vi "CSTK_BuildApplication_Manager_RenameEXEFileName.vi"(8 "错误输入（无错误）":errorcluster, 11 "BuildApplication Data in":T1={"Build Specification Name"="", "Destination Path"=path "", "Files Generated by Build"=[], "Exe Path Generated by Build"=path "", "Version"="", "Datatime"=timestamp(0 s since 1904-01-01), "ChangeLog"="", "Package as a ZIP file?"=TRUE, "Rename EXE File Name?"=FALSE, "Zip File Path"=path ""} {"Datatime" format="%<%.3X %x>T"}) -> (0 "错误输出":errorcluster, 3 "BuildApplication Data out":T1={"Build Specification Name"="", "Destination Path"=path "", "Files Generated by Build"=[], "Exe Path Generated by Build"=path "", "Version"="", "Datatime"=timestamp(0 s since 1904-01-01), "ChangeLog"="", "Package as a ZIP file?"=TRUE, "Rename EXE File Name?"=FALSE, "Zip File Path"=path ""} {"Datatime" format="%<%.3X %x>T"})   [LabVIEW 2015, in "CSTK_BuildApplication_Manager.lvlib"]
uses:
  CSTK_BuildApplication_Manager.lvlib
  CSTK_BuildApplication_Manager_data.ctl
  <userlib>/_OpenG.lib/array/array.llb/Delete Elements from 1D Array (Path)__ogtk.vi
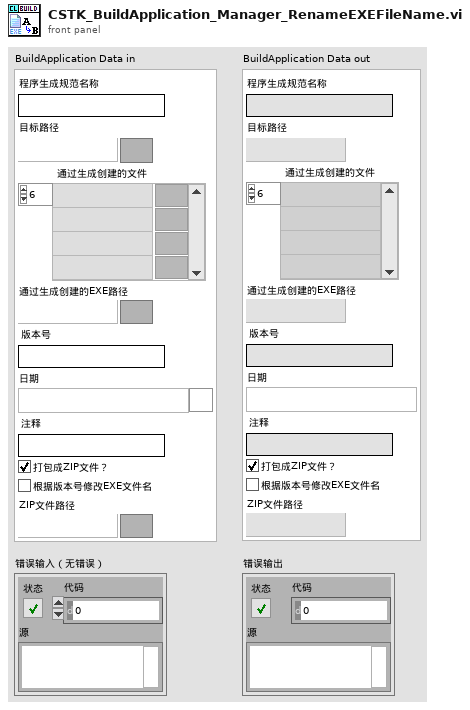
[diagram p1: front panel]
types:
  T1 = typedef "CSTK_BuildApplication_Manager.lvlib/CSTK_BuildApplication_Manager_data.ctl" = cluster{"Build Specification Name":string, "Destination Path":path, "Files Generated by Build":path[], "Exe Path Generated by Build":path, "Version":string, "Datatime":timestamp, "ChangeLog":string, "Package as a ZIP file?":bool, "Rename EXE File Name?":bool, "Zip File Path":path}
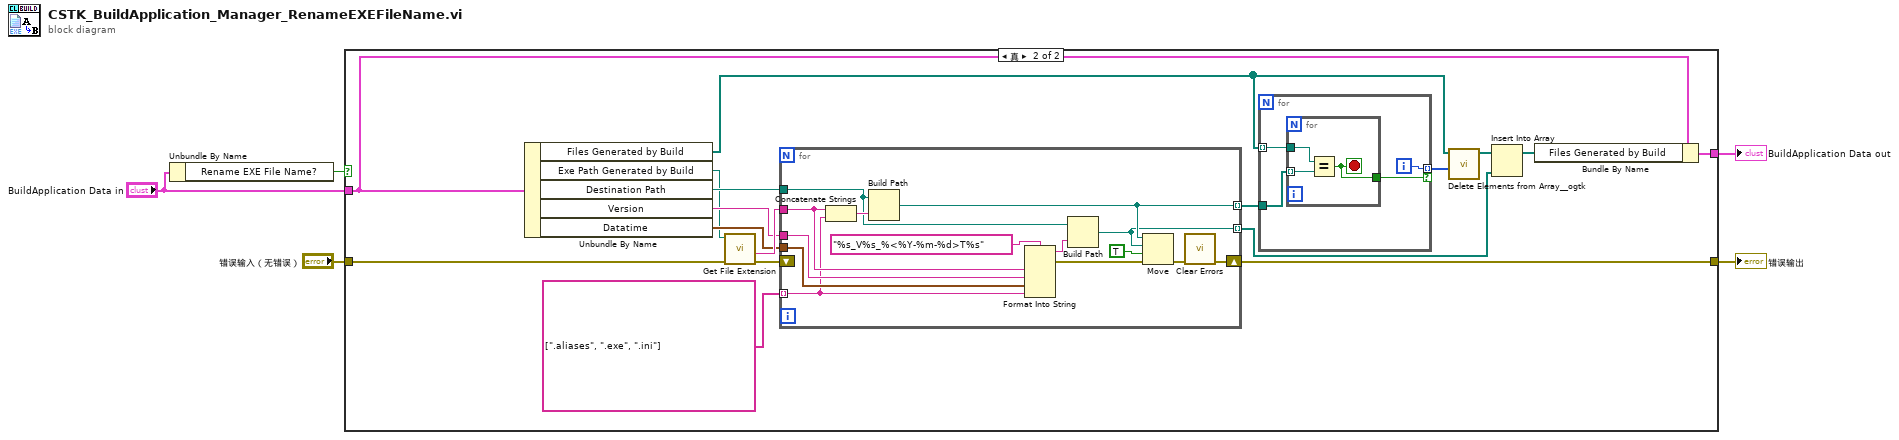
[diagram p0: block diagram]
diagram:
  n1 = Unbundle By Name("BuildApplication Data in") -> ("Rename EXE File Name?"=w3:bool)
  n2 = case shown="真" w3 {
    tunnel: "BuildApplication Data in" -> [w7 w12]
    tunnel: [w7 w10] -> w5
    tunnel: "错误输入（无错误）" -> [w6 w9]
    tunnel: [w6 w8] -> w1
    frame False {
    }
    frame True {
      n3 = Unbundle By Name(w12) -> ("Files Generated by Build"=w13:path[], "Exe Path Generated by Build"=w14:path, "Destination Path"=w15:path, "Version"=w17:string, "Datatime"=w16:timestamp)
      n4 = call <vilib>:"Get File Extension.vi"("error in (no error)"=w9, "file"=w14) -> ("error out"=w20:errorcluster, "filename without extension"=w19:string)  [unwired: 5 in, 3 out]
      n5 = for {
        tunnel: string[] [".aliases", ".exe", ".ini"] -> [w40] mode=indexing
        tunnel: w19 -> [w43]
        tunnel: w15 -> [w39]
        tunnel: w17 -> [w42]
        tunnel: w16 -> [w41]
        shift-right: [w34] -> w8
        shift-left: w20 -> [_]
        tunnel: [w33] -> w23 mode=indexing
        tunnel: [w32] -> w22 mode=indexing
        n6 = Concatenate Strings(w43, w40) -> (w45:string)
        n7 = Build Path(base path=w39, name or relative path=w45) -> (appended path=w33:path)
        n8 = Format Into String(format string="%s_V%s_%<%Y-%m-%d>T%s" ("格式字符串"), w43, w42, w41, w40) -> (resulting string=w38:string, error out=w36:errorcluster)  [unwired: 2 in]
        n9 = Build Path(base path=w39, name or relative path=w38) -> (appended path=w32:path)
        n10 = Move(source path=w33, error in=w36, 9:TRUE ("覆盖(F)"), 10:w32) -> (error out=w35:errorcluster)  [unwired: 1 in, 2 out]
        n11 = call <vilib>:"Clear Errors.vi"("error in (no error)"=w35) -> ("error out"=w34:errorcluster)  [unwired: 5 in, 1 out]
      }
      n12 = for {
        tunnel: w13 -> [w27] mode=indexing
        tunnel: w23 -> [w28]
        tunnel: [w26] -> w24 mode=indexing if=w25
        i -> [w26]
        n13 = for {
          tunnel: w28 -> [w30] mode=indexing
          tunnel: w27 -> [w31]
          tunnel: [w29] -> w25
          stop <- w29 stop-if-true
          n14 = Equal?(x=w31, y=w30) -> (x = y?=w29:bool)
        }
      }
      n15 = call-poly <userlib>:"Delete Elements from Array__ogtk.vi"("indices"=w24, "array"=w13) -> ("array w/ subset deleted"=w21:path[])  [unwired: 8 in, 1 out]
      n16 = Insert Into Array(array=w21, new element=w22) -> (w11:path[])  [unwired: 1 in]
      n17 = Bundle By Name(cluster=w12, "Files Generated by Build"=w11) -> (w10:T1)
    }
  }
  "BuildApplication Data out" <- w5
  "错误输出" <- w1
